vi "Property of node_0.vi"() -> ()   [LabVIEW 2015]
panel:
  in  "stop":bool
  in  "Tab Control":enum32{"Page 1", "Page 2"}(tab)
  in  "String":string
  out "String 2":string
  out "length":i32
  in  "Blinking":bool
  # "Length of string with Property of Node"
  # "Pardeep Kumar"
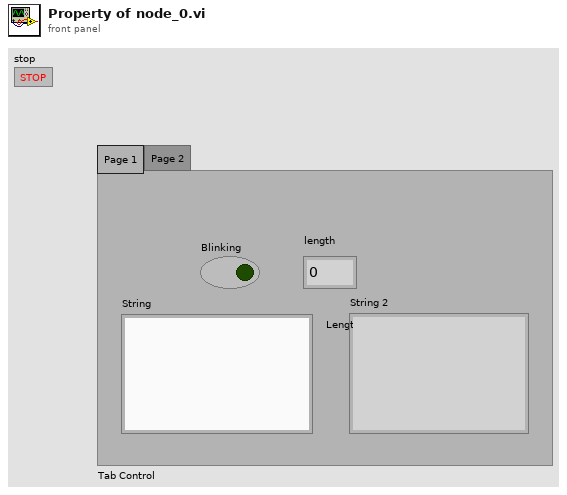
[diagram p1: front panel]
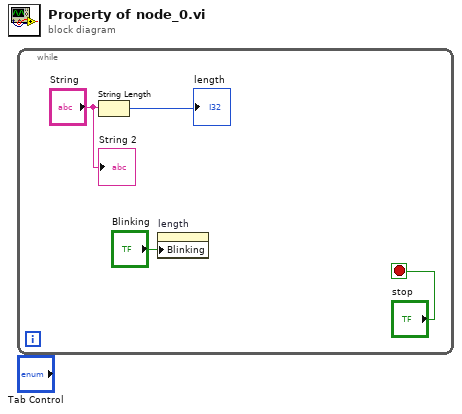
[diagram p0: block diagram]
diagram:
  n1 = while {
    stop <- "stop" stop-if-true
    n2 = String Length(string="String") -> (length=→"length":i32)
    n3 = property on="length" class="DigNum (strict)"("Blinking"="Blinking") -> ()  [unwired: 2 in, 2 out]
    "String 2" <- "String"
  }
